vi "MOVIE_save_path_definition.vi"(1 "Movie number":i32, 2 "Movie folder name":string) -> (0 "Movie path":path)   [LabVIEW 2015]
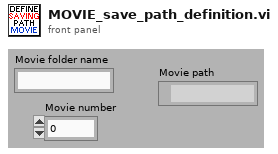
[diagram p1: front panel]
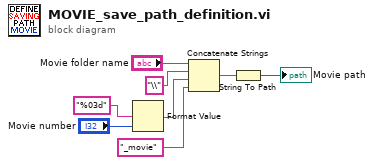
[diagram p0: block diagram]
diagram:
  n1 = Format Value(format string="%03d" ("string (\"\")"), value (0)="Movie number") -> (output string=w4:string)  [unwired: 1 in]
  n2 = Concatenate Strings("Movie folder name", "\\" ("string"), w4, "_movie" ("string")) -> (w6:string)
  n3 = String To Path(string=w6) -> (path=→"Movie path":path)
